vi "Setup DC Loads.vi"(8 "Error in":errorcluster caption="Error in (no error)", 10 "DC Loads":refnum<class "Instrument.lvclass">[](array[class]), 11 "Test Class in":refnum<class "Test Class.lvclass">) -> (0 "Error out":errorcluster)   [LabVIEW 2015, in "Instrument Setup.lvclass"]
uses:
  Instrument Setup.lvclass
  Classes/Instruments/Instrument/Class/Instrument.lvclass
  Test Class/Test Class.lvclass
  Classes/Instruments/DC Load/DC Load/Class/DC Load.lvclass
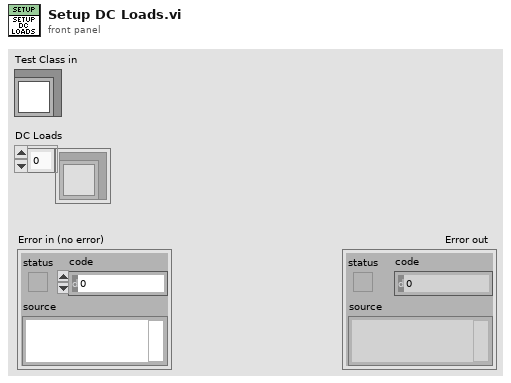
[diagram p1: front panel]
types:
  T1 = cluster{"Current":dbl, "Voltage":dbl, "LED VF":dbl, "RD Coeffecient":dbl, "LED Rd Ohm":dbl}
  T2 = cluster{"Resistance":dbl, "Rise Slew Rate (A/s)":dbl, "Fall Slew Rate (A/s)":dbl}
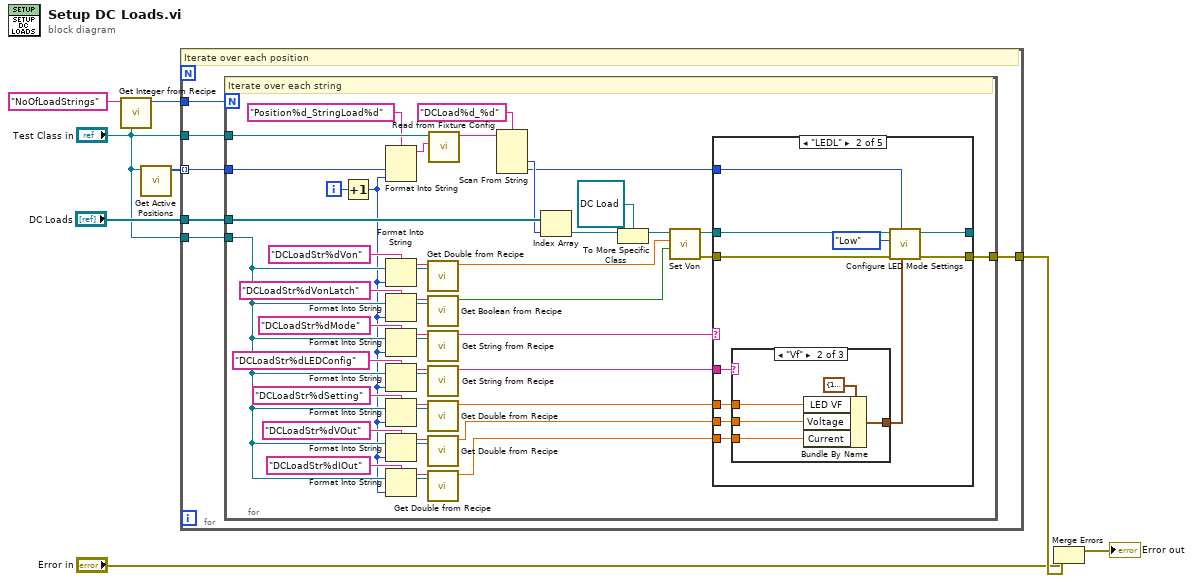
[diagram p0: block diagram]
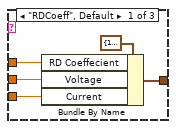
[diagram p3: hidden frame]
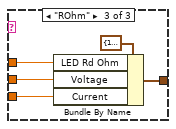
[diagram p4: hidden frame]
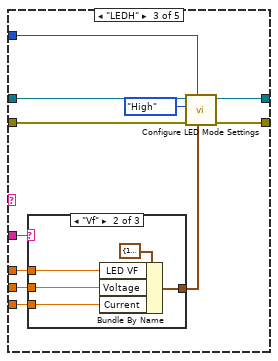
[diagram p5: hidden frame]
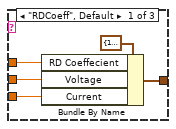
[diagram p6: hidden frame]
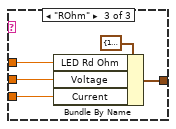
[diagram p7: hidden frame]
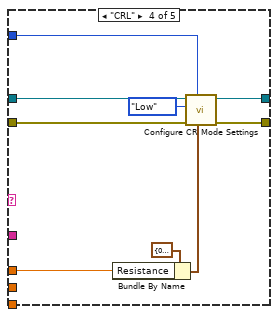
[diagram p8: hidden frame]
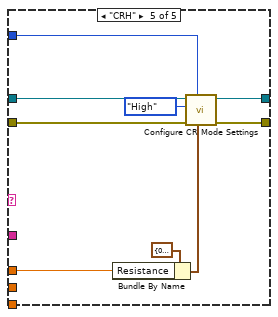
[diagram p9: hidden frame]
diagram:
  n1 = call "Get Integer from Recipe.vi"("Test Class in"="Test Class in", "Name"="NoOfLoadStrings" ("format string")) -> ("Value"=w2:i32)  [unwired: 7 in, 2 out]
  n2 = call "Get Active Positions.vi"("Test Class in"="Test Class in") -> ("Active Positions"=w5:u32[])  [unwired: 9 in, 1 out]
  n3 = for {
    tunnel: [w14] -> w7
    tunnel: w5 -> [w12] mode=indexing
    tunnel: "DC Loads" -> [w11]
    tunnel: "Test Class in" -> [w13]
    tunnel: w2 -> [w10]
    tunnel: "Test Class in" -> [w9]
    # "Iterate over each position"
    n4 = for {
      N: w10 -> [_]
      tunnel: [w49] -> w14
      tunnel: w13 -> [w48]
      tunnel: w12 -> [w47]
      tunnel: w11 -> [w43]
      tunnel: w9 -> [w37]
      i -> [w44]
      # "Iterate over each string"
      n5 = Increment(x=w44) -> (x+1=w15:i32)
      n6 = Format Into String(format string="Position%d_StringLoad%d", w47, w15) -> (resulting string=w46:string)  [unwired: 2 in, 1 out]
      n7 = Format Into String(format string="DCLoadStr%dVon" ("Name"), w15) -> (resulting string=w36:string)  [unwired: 2 in, 1 out]
      n8 = Format Into String(format string="DCLoadStr%dVonLatch" ("Name"), w15) -> (resulting string=w34:string)  [unwired: 2 in, 1 out]
      n9 = Format Into String(format string="DCLoadStr%dMode" ("Name"), w15) -> (resulting string=w31:string)  [unwired: 2 in, 1 out]
      n10 = Format Into String(format string="DCLoadStr%dLEDConfig" ("Name"), w15) -> (resulting string=w30:string)  [unwired: 2 in, 1 out]
      n11 = Format Into String(format string="DCLoadStr%dSetting" ("Name"), w15) -> (resulting string=w28:string)  [unwired: 2 in, 1 out]
      n12 = Format Into String(format string="DCLoadStr%dVOut" ("Name"), w15) -> (resulting string=w26:string)  [unwired: 2 in, 1 out]
      n13 = Format Into String(format string="DCLoadStr%dIOut" ("Name"), w15) -> (resulting string=w24:string)  [unwired: 2 in, 1 out]
      n14 = call "Get Double from Recipe.vi"("Test Class in"=w37, "Name"=w36) -> ("Value"=w22:dbl)  [unwired: 7 in, 2 out]
      n15 = call "Get Boolean from Recipe.vi"("Test Class in"=w37, "Name"=w34) -> ("Value"=w21:bool)  [unwired: 7 in, 2 out]
      n16 = call "Get String from Recipe.vi"("Test Class in"=w37, "Name"=w31) -> ("Value"=w20:string)  [unwired: 7 in, 2 out]
      n17 = call "Get String from Recipe.vi"("Test Class in"=w37, "Name"=w30) -> ("Value"=w19:string)  [unwired: 7 in, 2 out]
      n18 = call "Get Double from Recipe.vi"("Test Class in"=w37, "Name"=w28) -> ("Value"=w18:dbl)  [unwired: 7 in, 2 out]
      n19 = call "Get Double from Recipe.vi"("Test Class in"=w37, "Name"=w26) -> ("Value"=w17:dbl)  [unwired: 7 in, 2 out]
      n20 = call "Get Double from Recipe.vi"("Test Class in"=w37, "Name"=w24) -> ("Value"=w16:dbl)  [unwired: 7 in, 2 out]
      n21 = call-dynamic "Read from Fixture Config.vi"("Key"=w46, "Test Class in"=w48) -> ("Instrument Info"=w42:string)  [unwired: 8 in, 1 out]
      n22 = Scan From String(format string="DCLoad%d_%d", input string=w42) -> (output 1=w40:i32, output 2=w38:i32)  [unwired: 4 in, 3 out]
      n23 = Index Array(array=w43, index=w40) -> (element=w39:refnum<class "Instrument.lvclass">)
      n24 = To More Specific Class(target class=refnum<class "DC Load.lvclass"> refnum ("DC Load out"), reference=w39) -> (specific class reference=w51:refnum<class "DC Load.lvclass">)  [unwired: 1 in, 1 out]
      n25 = call-dynamic "Set Von.vi"("Von Latch"=w21, "Von"=w22, "DC Load in"=w51) -> ("error out"=w52:errorcluster, "DC Load out"=w53:refnum<class "DC Load.lvclass">)  [unwired: 7 in]
      n26 = case shown="\"LEDL\"" w20 {
        tunnel: w53 -> [w55 w66 w92 w116 w125]
        tunnel: w19 -> [_ w65 w91 _ _]
        tunnel: w18 -> [_ w63 w89 w114 w123]
        tunnel: w17 -> [_ w62 w88 _ _]
        tunnel: w16 -> [_ w61 w87 _ _]
        tunnel: [w54 w60 w86 w112 w121] -> w49
        tunnel: w52 -> [w54 w59 w85 w111 w120]
        tunnel: [w55 w58 w84 w110 w119] -> _
        tunnel: w38 -> [_ w56 w82 w108 w117]
        frame Default {
        }
        frame "LEDL" {
          n27 = case shown="\"Vf\"" w65 {
            tunnel: [w70 w75 w80] -> w64
            tunnel: w63 -> [w69 w74 w79]
            tunnel: w62 -> [w68 w73 w78]
            tunnel: w61 -> [w67 w72 w77]
            frame "RDCoeff", Default {
              n28 = Bundle By Name(cluster=T1 {"Current"=1.0, "Voltage"=1.5, "LED VF"=1.5, "RD Coeffecient"=1.0, "LED Rd Ohm"=100.0} ("LED Mode Settings"), "RD Coeffecient"=w69, "Voltage"=w68, "Current"=w67) -> (w70:T1)
            }
            frame "Vf" {
              n29 = Bundle By Name(cluster=T1 {"Current"=1.0, "Voltage"=1.5, "LED VF"=1.5, "RD Coeffecient"=1.0, "LED Rd Ohm"=100.0} ("LED Mode Settings"), "LED VF"=w74, "Voltage"=w73, "Current"=w72) -> (w75:T1)
            }
            frame "ROhm" {
              n30 = Bundle By Name(cluster=T1 {"Current"=1.0, "Voltage"=1.5, "LED VF"=1.5, "RD Coeffecient"=1.0, "LED Rd Ohm"=100.0} ("LED Mode Settings"), "LED Rd Ohm"=w79, "Voltage"=w78, "Current"=w77) -> (w80:T1)
            }
          }
          n31 = call-dynamic "Configure LED Mode Settings.vi"("LED Mode Settings"=w64, "Channel"=w56, "error in (no error)"=w59, "Range"=enum16{"High", "Low"}."Low", "DC Load in"=w66) -> ("error out"=w60:errorcluster, "DC Load out"=w58:refnum<class "DC Load.lvclass">)  [unwired: 5 in]
        }
        frame "LEDH" {
          n32 = case shown="\"Vf\"" w91 {
            tunnel: [w96 w101 w106] -> w90
            tunnel: w89 -> [w95 w100 w105]
            tunnel: w88 -> [w94 w99 w104]
            tunnel: w87 -> [w93 w98 w103]
            frame "RDCoeff", Default {
              n33 = Bundle By Name(cluster=T1 {"Current"=1.0, "Voltage"=1.5, "LED VF"=1.5, "RD Coeffecient"=1.0, "LED Rd Ohm"=100.0} ("LED Mode Settings"), "RD Coeffecient"=w95, "Voltage"=w94, "Current"=w93) -> (w96:T1)
            }
            frame "Vf" {
              n34 = Bundle By Name(cluster=T1 {"Current"=1.0, "Voltage"=1.5, "LED VF"=1.5, "RD Coeffecient"=1.0, "LED Rd Ohm"=100.0} ("LED Mode Settings"), "LED VF"=w100, "Voltage"=w99, "Current"=w98) -> (w101:T1)
            }
            frame "ROhm" {
              n35 = Bundle By Name(cluster=T1 {"Current"=1.0, "Voltage"=1.5, "LED VF"=1.5, "RD Coeffecient"=1.0, "LED Rd Ohm"=100.0} ("LED Mode Settings"), "LED Rd Ohm"=w105, "Voltage"=w104, "Current"=w103) -> (w106:T1)
            }
          }
          n36 = call-dynamic "Configure LED Mode Settings.vi"("LED Mode Settings"=w90, "Channel"=w82, "error in (no error)"=w85, "Range"=enum16{"High", "Low"}."High", "DC Load in"=w92) -> ("error out"=w86:errorcluster, "DC Load out"=w84:refnum<class "DC Load.lvclass">)  [unwired: 5 in]
        }
        frame "CRL" {
          n37 = Bundle By Name(cluster=T2 {"Resistance"=0.0, "Rise Slew Rate (A/s)"=0.04, "Fall Slew Rate (A/s)"=0.04} ("CR Mode Settings"), "Resistance"=w114) -> (w115:T2)
          n38 = call-dynamic "Configure CR Mode Settings.vi"("CR Mode Settings"=w115, "Channel"=w108, "error in (no error)"=w111, "Range"=enum16{"High", "Low"}."Low", "DC Load in"=w116) -> ("error out"=w112:errorcluster, "DC Load out"=w110:refnum<class "DC Load.lvclass">)  [unwired: 5 in]
        }
        frame "CRH" {
          n39 = Bundle By Name(cluster=T2 {"Resistance"=0.0, "Rise Slew Rate (A/s)"=0.04, "Fall Slew Rate (A/s)"=0.04} ("CR Mode Settings"), "Resistance"=w123) -> (w124:T2)
          n40 = call-dynamic "Configure CR Mode Settings.vi"("CR Mode Settings"=w124, "Channel"=w117, "error in (no error)"=w120, "Range"=enum16{"High", "Low"}."High", "DC Load in"=w125) -> ("error out"=w121:errorcluster, "DC Load out"=w119:refnum<class "DC Load.lvclass">)  [unwired: 5 in]
        }
      }
    }
  }
  n41 = Merge Errors("Error in", w7) -> (→"Error out":errorcluster)
